vi "M686 Position AE.vi"(1 "Position In":dbl[](array[numeric]), 2 "Action":T1) -> (0 "Position Out":dbl[](array[numeric]))   [LabVIEW 2014]
uses:
  Focus Lock/Controls/Standard Action for Focus Lock.ctl
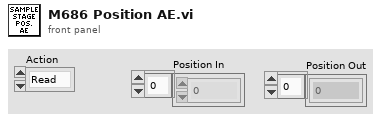
[diagram p1: front panel]
types:
  T1 = typedef "Standard Action for Focus Lock.ctl" = enum16{"Read", "Write"}
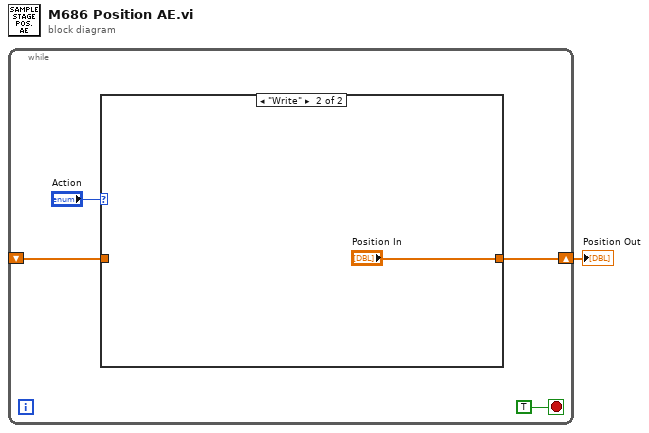
[diagram p0: block diagram]
diagram:
  n1 = while {
    shift-right: [w3] -> w1
    shift-left: _ -> [w2]
    stop <- TRUE stop-if-true
    n2 = case shown="\"Write\"" "Action" {
      tunnel: [w6 "Position In"] -> w3
      tunnel: w2 -> [w6 _]
      frame "Read", Default {
      }
      frame "Write" {
      }
    }
  }
  "Position Out" <- w1
